vi "Write loop condition.vi"(5 "conditional terminal":refnum<class "Terminal.lvclass">, 9 "Loop in":refnum<class "Loop.lvclass">) -> (3 "Loop out":refnum<class "Loop.lvclass">)   [LabVIEW 2014, in "Loop.lvclass"]
uses:
  Loop.lvclass
  Terminal/Terminal.lvclass
  Loop.lvclass/Loop.ctl
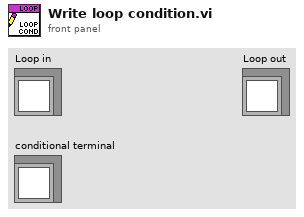
[diagram p1: front panel]
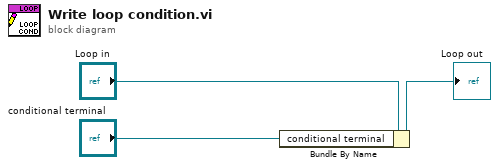
[diagram p0: block diagram]
diagram:
  n1 = Bundle By Name(cluster="Loop in", "conditional terminal"="conditional terminal") -> (→"Loop out":refnum<class "Loop.lvclass">)
